vi "Email Loop.vi"   [LabVIEW 2019]
uses:
  Controls/Email Mode.ctl
types:
  T1 = typedef "Email Mode.ctl" = enum16{"Trigger Email", "Send Email"}
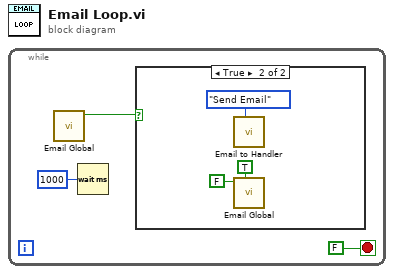
[diagram p0: block diagram]
diagram:
  n1 = while {
    stop <- FALSE stop-if-true
    n2 = call "Email Global.vi"() -> ("Send Email OUT"=w1:bool)  [unwired: 11 in]
    n3 = Wait (ms)(milliseconds to wait=u32 1000) -> ()  [unwired: 1 out]
    n4 = case shown="True" w1 {
      frame False {
      }
      frame True {
        n5 = call "Email to Handler.vi"("Email Mode"=Email_Mode."Send Email") -> ()  [unwired: 11 in]
        n6 = call "Email Global.vi"("Write (F)"=TRUE, "Send Email"=FALSE) -> ()  [unwired: 9 in, 1 out]
      }
    }
  }
